vi "Set Initialization Data - DataLog.vi"(8 "error in":errorcluster, 11 "Maestro Control in":refnum<class "Maestro Control.lvclass">) -> (0 "error out":errorcluster, 3 "Maestro Control out":refnum<class "Maestro Control.lvclass">)   [LabVIEW 2021, in "Maestro Control.lvclass"]
doc: "Sets the initialization data of a statically linked subWorker."
uses:
  Maestro Control.lvclass
  Maestro Data Logg/Initialization Data.ctl
  Maestro Control.lvclass/Maestro Control.ctl
  Maestro Data Logg/Maestro Data Logg.lvclass
  C:/Program Files (x86)/National Instruments/LabVIEW 2021/vi.lib/addons/_Workers/Library/Classes/Worker/Worker.lvclass
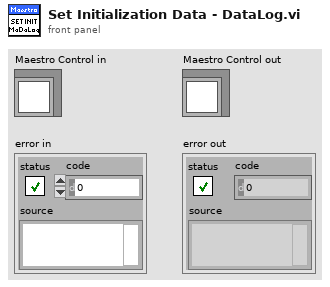
[diagram p1: front panel]
types:
  T1 = typedef "Maestro Data Logg.lvclass/Initialization Data.ctl" = cluster{"String":string, "Data Queue":refnum<queue>}
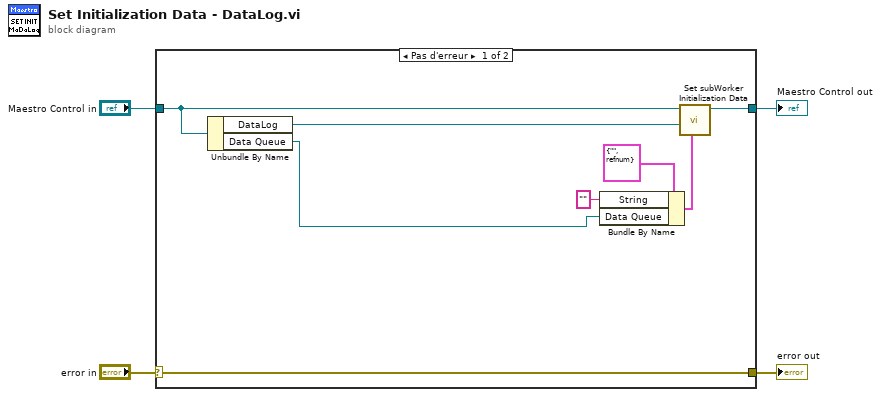
[diagram p0: block diagram]
diagram:
  n1 = case shown="Pas d'erreur" "error in" {
    selector: "error in" -> [w12 w14]
    tunnel: [w12 w14] -> w3
    tunnel: [w10 w13] -> w2
    tunnel: "Maestro Control in" -> [w9 w13]
    frame No Error {
      n2 = Unbundle By Name(w9) -> ("DataLog"=w11:refnum<class "Maestro Data Logg.lvclass">, "Data Queue"=w5:refnum<queue>)
      n3 = Bundle By Name(cluster=T1 {"String"="", "Data Queue"=refnum} ("Initialization Data"), "String"="" ("Placeholder"), "Data Queue"=w5) -> (w7:T1)
      n4 = call-dynamic "Set subWorker Initialization Data.vi"("Initialization Data"=w7, "subWorker"=w11, "Worker"=w9) -> ("Worker out"=w10:refnum<class "Maestro Control.lvclass">)  [unwired: 8 in]
    }
    frame Error {
    }
  }
  "error out" <- w3
  "Maestro Control out" <- w2
